vi "String to JSON Value.vi"(1 "Value":string="world", 2 "Name":string="hello") -> (0 "JSON Value":string)   [LabVIEW 2011, in "LV JSON.lvlib"]
uses:
  LV JSON.lvlib
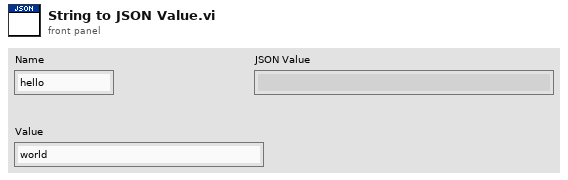
[diagram p1: front panel]
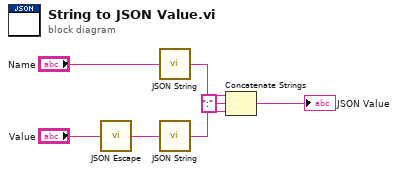
[diagram p0: block diagram]
diagram:
  n1 = call "JSON Escape.vi"("JSON String"="Value") -> ("Escaped JSON String"=w1:string)
  n2 = call "JSON String.vi"("in"="Name") -> ("out"=w6:string)
  n3 = call "JSON String.vi"("in"=w1) -> ("out"=w5:string)
  n4 = Concatenate Strings(w6, ":" ("string"), w5) -> (→"JSON Value":string)
